vi "InitAction.vi"(6 "InstrumentName":string, 7 "VisaRessIn":refnum<visa-resource-name>, 8 "error in (no error)":errorcluster caption="entrée d'erreur (pas d'erreur)", 9 "FirstClassInst":bool, 10 "Function":string, 11 "GenData In":refnum<class "MultiHarp150.lvclass"> caption="DNL_LabVIEW Object in") -> (0 "error out":errorcluster caption="sortie d'erreur", 3 "GenData Out":refnum<class "MultiHarp150.lvclass"> caption="DNL_LabVIEW Object out")   [LabVIEW 2019, in "MultiHarp150.lvclass"]
uses:
  MultiHarp150.lvclass
  MultiHarp150_Func.ctl
  MultiHarp150.lvclass/MultiHarp150.ctl
  <userlib>/MultiHarp150/MH_DllPath_global.vi
panel:
  in  "DefaultDev_Func":T1
  out "VisaRessOut":refnum<visa-resource-name>
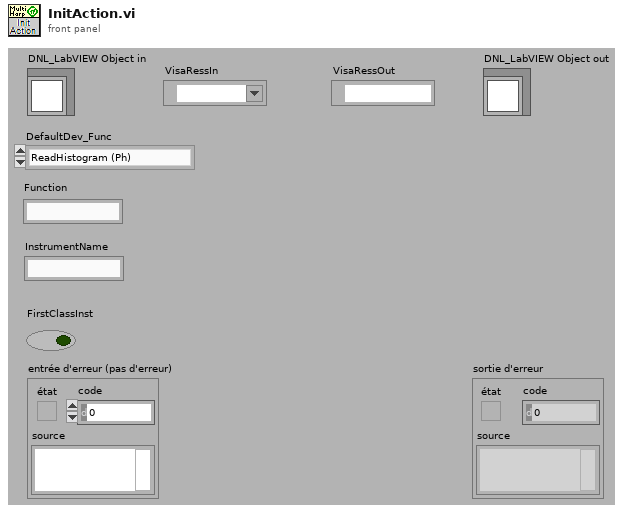
[diagram p1: front panel]
types:
  T1 = typedef "MultiHarp150.lvclass/MultiHarp150_Func.ctl" = enum16{"ReadHistogram (Ph)", "ReadCount (Ph)"}
  T2 = enum16{"1024", "2048", "4096", "8192", "16384", "32768", "65536"}
  T3 = enum16{"5", "10", "20", "40", "80", "160", "320", "640", "1280", "2560", "5120", "10240", "20480", "40960", "81920", "163840", "327680", "655360", "1310720", "2621440", "5242880", "10485760", "20971520", "41943040"}
  T4 = typedef "MH_InputChannel_LS.ctl" = cluster{"Name":string, "Enable":bool, "Edge":i32, "Level":i32, "Offset":i32, "UseDeadTime":bool, "DeadTime":i32}
  T5 = typedef "MH_MeasMode.ctl" = i32
  T6 = typedef "MH_RefSource.ctl" = enum16{"INTERNAL", "EXTERNAL_10MHZ", "WR_MASTER_GENERIC", "WR_SLAVE_GENERIC", "WR_GRANDM_GENERIC", "EXTN_GPS_PPS", "EXTN_GPS_PPS_UART", "WR_MASTER_MHARP", "WR_SLAVE_MHARP", "WR_GRANDM_MHARP"}
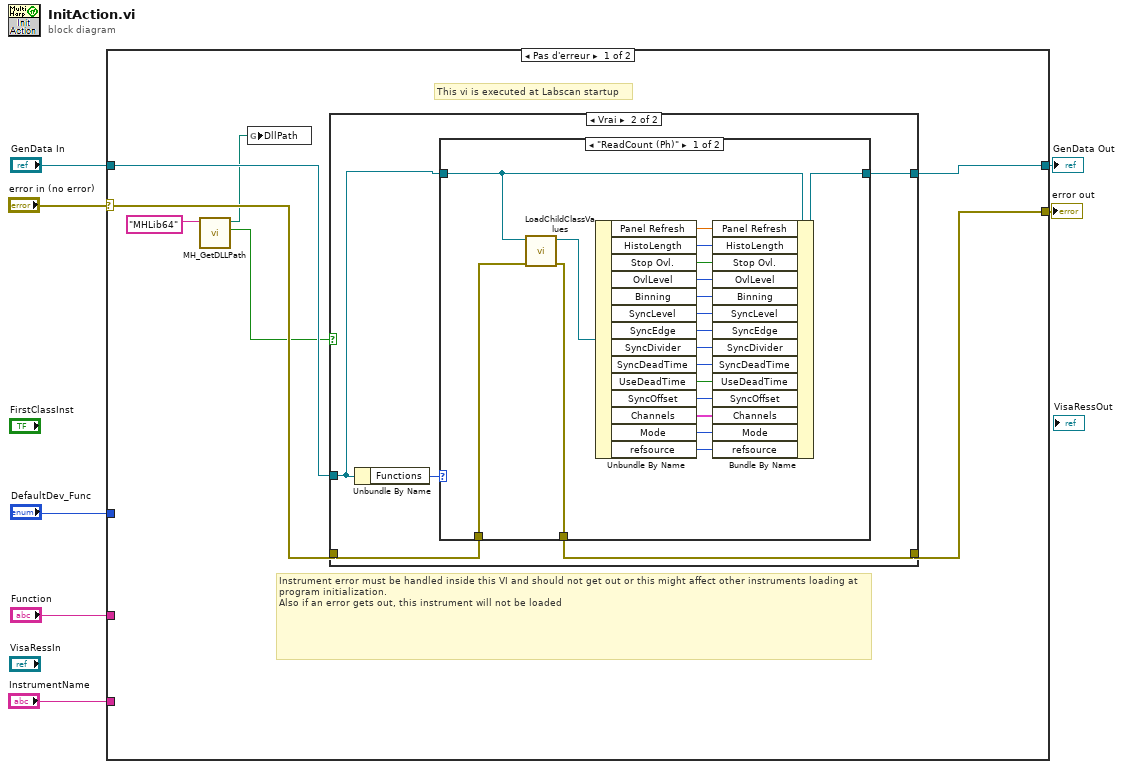
[diagram p0: block diagram]
diagram:
  n1 = case shown="Pas d'erreur" "error in (no error)" {
    selector: "error in (no error)" -> [w10 w44]
    tunnel: [w12 w44] -> w6
    tunnel: "GenData In" -> [w14 w43]
    tunnel: [w13 w43] -> w4
    tunnel: "DefaultDev_Func" -> [_ _]
    tunnel: "Function" -> [_ _]
    tunnel: "InstrumentName" -> [_ _]
    frame No Error {
      # "This vi is executed at Labscan startup"
      # "Instrument error must be handled inside this VI and should not get out or this might affect other instruments loading at program initialization.\nAlso if an error gets out, this instrument will not be loaded"
      n2 = call <userlib>:"MH_GetDLLPath.vi"("DllName_64bit"="MHLib64" ("name or relative path")) -> ("file exists?"=w9:bool, "DLLPath"=w8:path)  [unwired: 9 in]
      n3 = global write "MH_DllPath_global.vi" "DllPath"(w8) -> ()
      n4 = case shown="Vrai" w9 {
        tunnel: w14 -> [w16 w20]
        tunnel: [w16 w19] -> w13
        tunnel: [w15 w18] -> w12
        tunnel: w10 -> [w15 w17]
        frame False {
        }
        frame True {
          n5 = Unbundle By Name(w20) -> ("Functions"=w21:T1)
          n6 = case shown="\"ReadCount (Ph)\"" w21 {
            tunnel: w20 -> [w40 w42]
            tunnel: [w39 w42] -> w19
            tunnel: w17 -> [w37 w41]
            tunnel: [w36 w41] -> w18
            frame "ReadCount (Ph)" {
              n7 = call "LoadChildClassValues.vi"("error in (no error)"=w37, "MultiHarp150 en entrée"=w40) -> ("error out"=w36:errorcluster, "MultiHarp150 en sortie"=w38:refnum<class "MultiHarp150.lvclass">)  [unwired: 8 in]
              n8 = Unbundle By Name(w38) -> ("Panel Refresh"=w35:dbl, "HistoLength"=w34:T2, "Stop Ovl."=w33:bool, "OvlLevel"=w32:u32, "Binning"=w31:T3, "SyncLevel"=w30:i32, "SyncEdge"=w29:i32, "SyncDivider"=w28:i32, "SyncDeadTime"=w27:i32, "UseDeadTime"=w26:bool, "SyncOffset"=w25:i32, "Channels"=w24:T4[], "Mode"=w23:T5, "refsource"=w22:T6)
              n9 = Bundle By Name(cluster=w40, "Panel Refresh"=w35, "HistoLength"=w34, "Stop Ovl."=w33, "OvlLevel"=w32, "Binning"=w31, "SyncLevel"=w30, "SyncEdge"=w29, "SyncDivider"=w28, "SyncDeadTime"=w27, "UseDeadTime"=w26, "SyncOffset"=w25, "Channels"=w24, "Mode"=w23, "refsource"=w22) -> (w39:refnum<class "MultiHarp150.lvclass">)
            }
            frame Default {
            }
          }
        }
      }
    }
    frame Error {
    }
  }
  "error out" <- w6
  "GenData Out" <- w4
